vi "Variant_BuildClusterFromElementArray.vi"(9 "name":string, 10 "Elements":variant[](array[variant])) -> (3 "Cluster":variant)   [LabVIEW 2017, in "JSONtext.lvlib"]
uses:
  JSONtext.lvlib
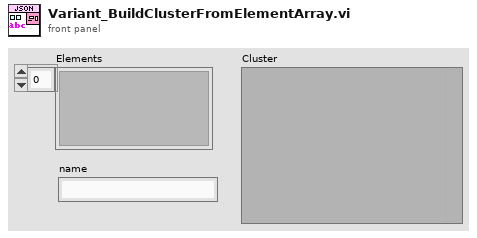
[diagram p1: front panel]
types:
  T1 = typedef "Type Descriptor I16 Array.ctl" = T2[]
  T2 = typedef "Type Descriptor I16.ctl" = i16
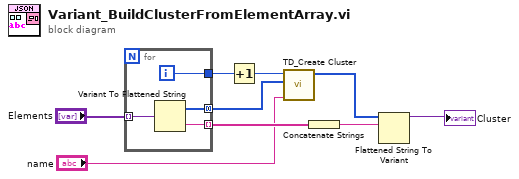
[diagram p0: block diagram]
diagram:
  n1 = for {
    tunnel: "Elements" -> [w13] mode=indexing
    tunnel: [w12] -> w1 mode=concatenating
    tunnel: [w11] -> w8 mode=indexing
    tunnel: [w10] -> w5
    i -> [w10]
    n2 = Variant To Flattened String(Variant=w13) -> (data string=w11:string, 1:w12:i16[])
  }
  n3 = Increment(x=w5) -> (x+1=w4:i32)
  n4 = call <vilib>:"TD_Create Cluster.vi"("Name"="name", "Concatenated Elts"=w1, "N Elts"=w4) -> ("ClusterTD"=w2:T1)  [unwired: 8 in]
  n5 = Concatenate Strings(w8) -> (w9:string)
  n6 = Flattened String To Variant(6:w9, 7:w2) -> (3:→"Cluster":variant)  [unwired: 1 in, 1 out]
